vi "create weights.vi"(0 "Input":dbl[][](array[numeric])=[[1.0, -1.0, 1.5, -1.3, -0.5], [1.0, 1.0, 1.2, 1.2, 0.7], [1.0, 1.0, 0.9, 0.5, 0.8]], 1 "Target Output":dbl[][](array[numeric])=[[1.0, 0.0, 1.0, 0.0, 0.0], [0.0, 1.0, 0.0, 1.0, 1.0]], 2 "Number of Hidden Neurons":i32(slide)=6 scale=0.0..10.0, 3 "Learning Rate":dbl(slide)=0.49999999999999994 scale=0.0..1.0, 4 "Beta":dbl(slide)=1.0 scale=0.0..4.0) -> (5 "Weights 1":dbl[][](array[numeric]), 6 "Weights 2":dbl[][](array[numeric]), 7 "Error":dbl(graph))   [LabVIEW 2009]
panel:
  in  "stop":bool
  # "each column corresponds to an input/output pair"
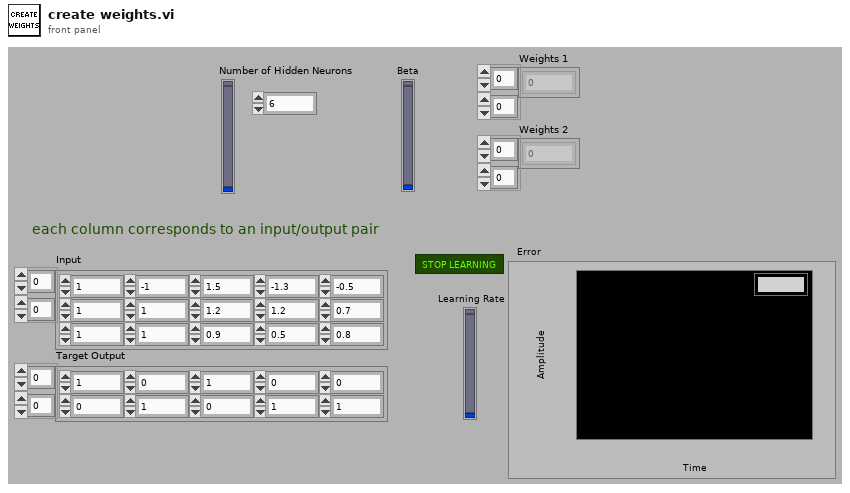
[diagram p1: front panel]
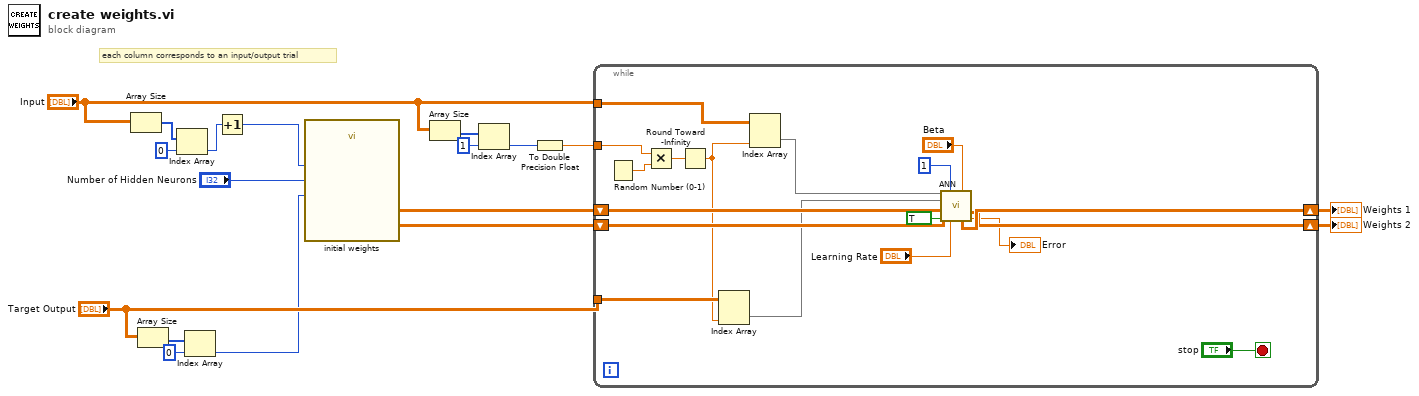
[diagram p0: block diagram]
diagram:
  # "each column corresponds to an input/output trial"
  n1 = Array Size(array="Input") -> (size(s)=w14:i32[])
  n2 = Array Size(array="Target Output") -> (size(s)=w5:i32[])
  n3 = Index Array(array=w14, index=0) -> (element=w12:i32)
  n4 = Index Array(array=w5, index=0) -> (element=w3:i32)
  n5 = Increment(x=w12) -> (x+1=w18:i32)
  n6 = call "initial weights.vi"("Number of classifiers"=w3, "Number of hidden neurons"="Number of Hidden Neurons", "Inputs + 1"=w18) -> ("Weights 2"=w15:dbl[][], "Weights 1"=w16:dbl[][])
  n7 = Array Size(array="Input") -> (size(s)=w10:i32[])
  n8 = Index Array(array=w10, index=1) -> (element=w8:i32)
  n9 = To Double Precision Float(number=w8) -> (double precision float=w7:dbl)
  n10 = while {
    tunnel: "Input" -> [w29]
    shift-right: [w32] -> w2
    shift-left: w16 -> [w34]
    shift-right: [w31] -> w1
    shift-left: w15 -> [w33]
    tunnel: w7 -> [w27]
    tunnel: "Target Output" -> [w25]
    stop <- "stop" stop-if-true
    n11 = Random Number (0-1)() -> (number: 0 to 1=w28:dbl)
    n12 = Multiply(x=w27, y=w28) -> (x*y=w22:dbl)
    n13 = Round Toward -Infinity(1:w22) -> (0:w21:dbl)
    n14 = Index Array(array=w25, index (col)=w21) -> (element=w24:dbl[])  [unwired: 1 in]
    n15 = Index Array(array=w29, index (col)=w21) -> (element=w26:dbl[])  [unwired: 1 in]
    n16 = call "ANN.vi"("Input"=w26, "Iterations"=1, "Beta"="Beta", "Target Output"=w24, "Weight_2"=w33, "Weight_1"=w34, "Back Propagation"=TRUE, "Learning Rate"="Learning Rate") -> ("Weight_2_out"=w31:dbl[][], "Weight_1_out"=w32:dbl[][], "Error"=→"Error":dbl)  [unwired: 4 in, 1 out]
  }
  "Weights 1" <- w2
  "Weights 2" <- w1
